vi "fpga_LP2 Filter_coefblock (M Class_50Hz).vi"(0 "Memory In":refnum<k21>="coefROM", 2 "coefAddr":fxp<+,10,10>) -> (7 "coefficients":fxp<+/-,19,-3>[](array[numeric]) format="%#.16g", 9 "error":i32)   [LabVIEW 2013, in "NI_EP_PMU_FPGA.lvlib"]
uses:
  <vilib>/addons/Electrical Power/PMU/NI_EP_PMU_FPGA.lvlib
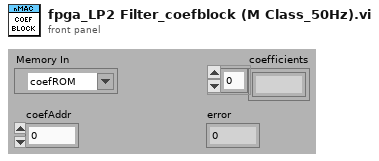
[diagram p1: front panel]
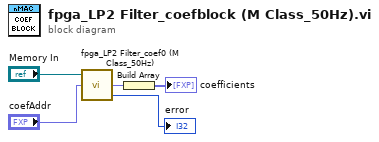
[diagram p0: block diagram]
diagram:
  n1 = call <vilib>:"fpga_LP2 Filter_coef0 (M Class_50Hz).vi"("Memory In"="Memory In", "coefAddr"="coefAddr") -> ("coef"=w4:fxp<+/-,19,-3>, "error"=→"error":i32)  [unwired: 6 in]
  n2 = Build Array ("MergeCoef")(w4) -> (→"coefficients":fxp<+/-,19,-3>[])
